vi "Find Class by Name.vi"(8 "error in (no error)":errorcluster, 10 "Name":string, 11 "Installed Instruments":refnum<class "Instrument.lvclass">[](array[class])) -> (0 "error out":errorcluster, 3 "Instrument out":refnum<class "Instrument.lvclass">)   [LabVIEW 2019, in "Control Experiment.lvclass"]
uses:
  Control Experiment.lvclass
  <userlib>/LevyLab/Instrument Framework/SMOs/Instrument/Instrument.lvclass
panel:
  out "Array":bool[](array[boolean])
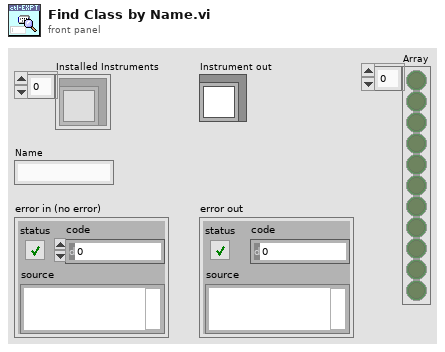
[diagram p1: front panel]
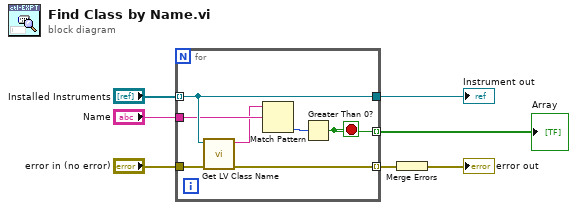
[diagram p0: block diagram]
diagram:
  n1 = for {
    tunnel: "Installed Instruments" -> [w13] mode=indexing
    tunnel: "Name" -> [w12]
    tunnel: [w13] -> w3
    tunnel: "error in (no error)" -> [w11]
    tunnel: [w10] -> w6 mode=indexing
    tunnel: [w8] -> w1 mode=indexing
    stop <- w8 stop-if-true
    n2 = call <vilib>:"Get LV Class Name.vi"("error in (no error)"=w11, "object"=w13) -> ("error out"=w10:errorcluster, "class name"=w9:string)  [unwired: 8 in]
    n3 = Match Pattern(string=w9, regular expression=w12) -> (offset past match=w14:i32)  [unwired: 1 in, 3 out]
    n4 = Greater Than 0?(x=w14) -> (x > 0?=w8:bool)
  }
  "Instrument out" <- w3
  "Array" <- w1
  n5 = Merge Errors(w6) -> (→"error out":errorcluster)
